vi "Build Internal State String.vi"(5 "State":string, 7 "Arguments (\"\")":string, 9 "Arg-State (\"\")":string, 11 "Source (\"\")":string) -> (6 "State with Arguments":string)   [LabVIEW 2014, in "JKI-State-Machine-Plus.lvlib"]
doc: "Builds a state string that contains arguments for the JKI State Machine.\n<B>For Example:</B> If State = A and Arguments = B then State with Arguments = A >> B\n\nFor instructions on how to use the JKI State Machine, examples and video tutorials, visit:\nhttp://jkisoft.com/state-machine/\n\n<B>Inputs:</B>\n <B>State:</B> The State string that requires the argument.\n <B>Arguments:</B> The Argument string to add to the state. The default is an empty string. If Argument is an empty string then State will be returned to the output. <B>Note:</B> The arguments input must not contain any unprintable characters like linefeed or carriage return.\n\n<B>Outputs:</B>\n <B>State with Arguments:</B> This output returns the new string that contains the State and the Argument. <B>For Example:</B> If State = A and Arguments = B then State with Arguments = A >> B\n\nJKI State Machine™ 2018.0.7.45\nhttp://jki.net/state-machine/\nCopyright (C) 2005-2018, JKI <info@jki.net>\nALL RIGHTS RESERVED"
uses:
  JKI-State-Machine-Plus.lvlib
panel:
  # "For instructions on how to use the JKI State Machine, examples and video tutorials, visit:\nhttp://jki.net/state-machine/\n\nJKI State Machine™\nhttp://jki.net/state-machine/\nCopyright (C) 2005-2017, JKI <info@jki.net>\nALL RIGHTS RESERVED"
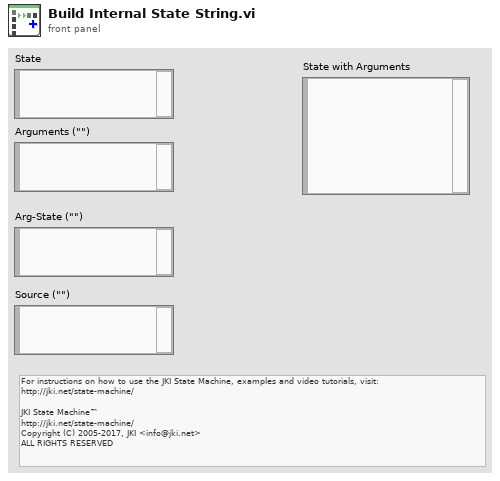
[diagram p1: front panel]
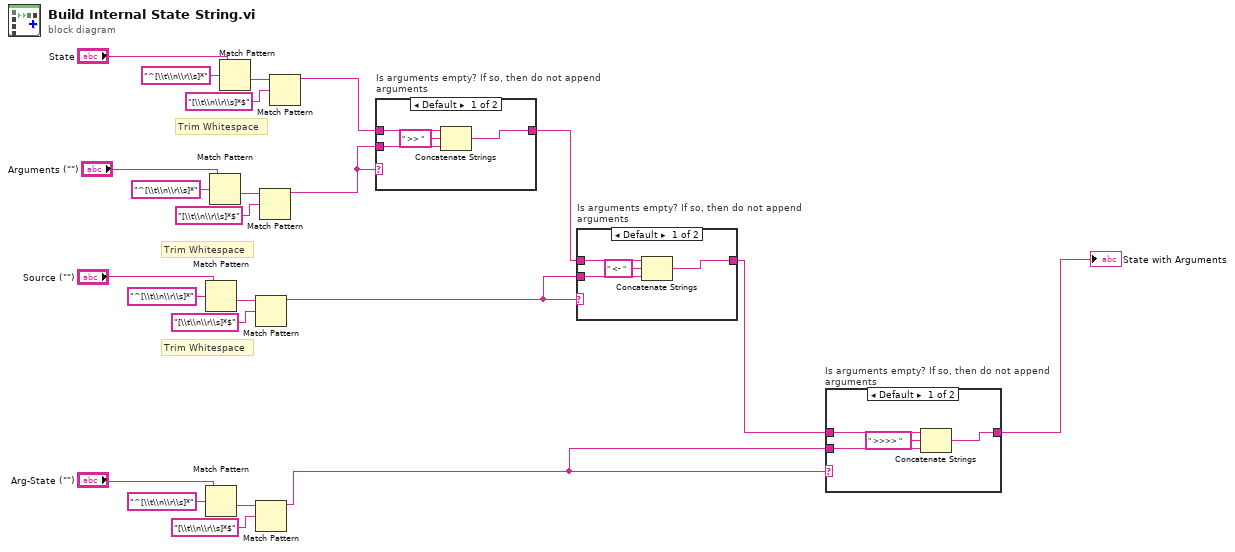
[diagram p0: block diagram]
diagram:
  # "Trim Whitespace"
  # "Trim Whitespace"
  # "Trim Whitespace"
  n1 = Match Pattern(string="Source (\"\")", regular expression="^[\\t\\n\\r\\s]*") -> (after substring=w12:string)  [unwired: 1 in, 3 out]
  n2 = Match Pattern(string="Arg-State (\"\")", regular expression="^[\\t\\n\\r\\s]*") -> (after substring=w7:string)  [unwired: 1 in, 3 out]
  n3 = Match Pattern(string="Arguments (\"\")", regular expression="^[\\t\\n\\r\\s]*") -> (after substring=w17:string)  [unwired: 1 in, 3 out]
  n4 = Match Pattern(string="State", regular expression="^[\\t\\n\\r\\s]*") -> (after substring=w22:string)  [unwired: 1 in, 3 out]
  n5 = Match Pattern(string=w12, regular expression="[\\t\\n\\r\\s]*$") -> (before substring=w9:string)  [unwired: 1 in, 3 out]
  n6 = Match Pattern(string=w7, regular expression="[\\t\\n\\r\\s]*$") -> (before substring=w4:string)  [unwired: 1 in, 3 out]
  n7 = Match Pattern(string=w17, regular expression="[\\t\\n\\r\\s]*$") -> (before substring=w14:string)  [unwired: 1 in, 3 out]
  n8 = Match Pattern(string=w22, regular expression="[\\t\\n\\r\\s]*$") -> (before substring=w19:string)  [unwired: 1 in, 3 out]
  n9 = case "Is arguments empty? If so, then do not append arguments" shown="Default" w14 {
    tunnel: [w24 w28] -> w3
    tunnel: w19 -> [w27 w28]
    tunnel: w14 -> [w25 _]
    frame Default {
      n10 = Concatenate Strings(w27, " >> " ("string"), w25) -> (w24:string)
    }
    frame "" {
    }
  }
  n11 = case "Is arguments empty? If so, then do not append arguments" shown="Default" w9 {
    tunnel: [w29 w33] -> w2
    tunnel: w3 -> [w32 w33]
    tunnel: w9 -> [w30 _]
    frame Default {
      n12 = Concatenate Strings(w32, " <- " ("string"), w30) -> (w29:string)
    }
    frame "" {
    }
  }
  n13 = case "Is arguments empty? If so, then do not append arguments" shown="Default" w4 {
    tunnel: [w35 w38] -> w1
    tunnel: w2 -> [w37 w38]
    tunnel: w4 -> [w36 _]
    frame Default {
      n14 = Concatenate Strings(w37, " >>>> " ("string"), w36) -> (w35:string)
    }
    frame "" {
    }
  }
  "State with Arguments" <- w1
